vi "Get Names String.vi"(8 "error in (no error)":errorcluster, 11 "Array":refnum<vi>[](array[refnum])) -> (0 "error out":errorcluster, 3 "regular expression":string)   [LabVIEW 2025, in "Scripting Server.lvlib" / "Tools.lvlib"]
uses:
  Tools.lvlib
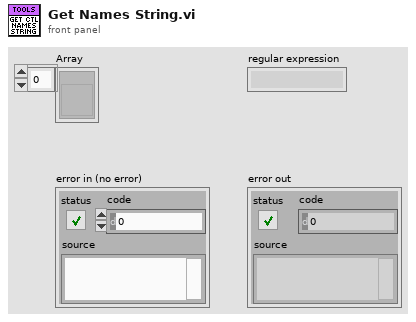
[diagram p1: front panel]
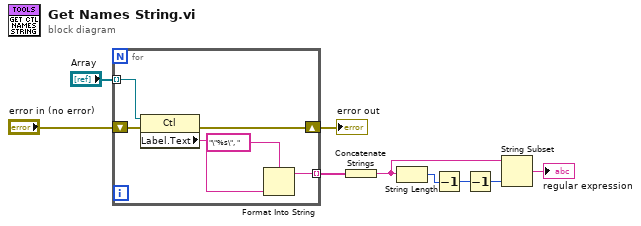
[diagram p0: block diagram]
diagram:
  n1 = for {
    tunnel: "Array" -> [w13] mode=indexing
    shift-right: [w14] -> w8
    shift-left: "error in (no error)" -> [w15]
    tunnel: [w10] -> w6 mode=indexing
    n2 = property class="Ctl"(reference=w13, error in=w15) -> (error out=w14:errorcluster, "Label.Text"=w12:string)  [unwired: 1 out]
    n3 = Format Into String(format string="\"%s\", ", w12) -> (resulting string=w10:string)  [unwired: 2 in, 1 out]
  }
  "error out" <- w8
  n4 = Concatenate Strings(w6) -> (w2:string)
  n5 = String Length(string=w2) -> (length=w4:i32)
  n6 = Decrement(x=w4) -> (x-1=w5:i32)
  n7 = Decrement(x=w5) -> (x-1=w3:i32)
  n8 = String Subset(string=w2, length (rest)=w3) -> (substring=→"regular expression":string)  [unwired: 1 in]
